vi "test_serial-w-arduino-1.vi"() -> ()   [LabVIEW 2019]
uses:
  <vilib>/Instr/_visa.llb/VISA Configure Serial Port (Instr).vi
panel:
  in  "s":bool
  in  "steer":u8(slide)=28 scale=15.0..35.0
  in  "dt":u32=50
  out "read buffer":string
  out "Numeric":i32
  out "Waveform Chart":u32(graph)
  in  "speed":u8(slide)=28 scale=1.0..255.0
  in  "write":bool
  in  "baud rate":u32=115200
  out "String":string
  in  "stop":bool
  out "write buffer":string
  in  "VISA resource name":refnum<visa-resource-name>="COM6"
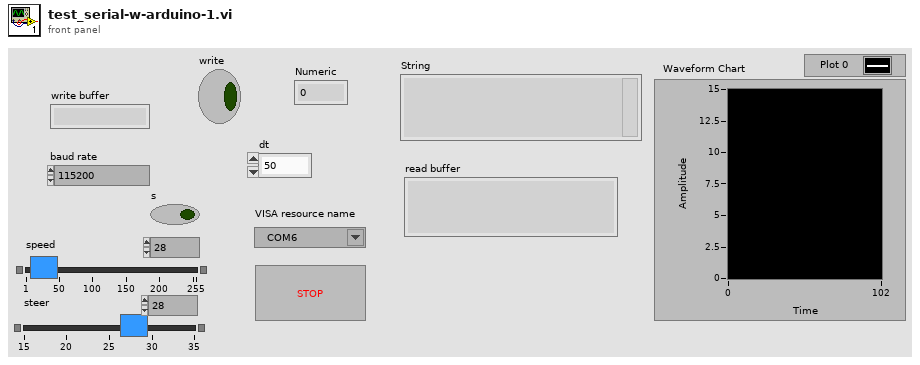
[diagram p1: front panel]
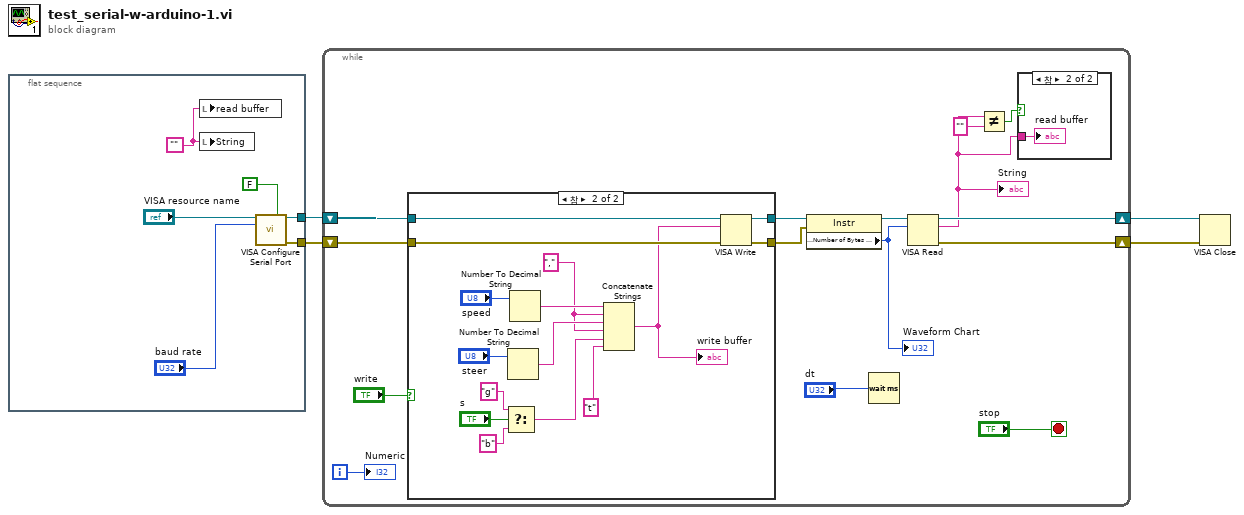
[diagram p0: block diagram]
diagram:
  n1 = flat-sequence {
    tunnel: [w9] -> w4
    tunnel: [w8] -> w1
    frame #0 {
      w5 = ""
      n2 = local write "read buffer"(w5) -> ()
      n3 = local write "String"(w5) -> ()
      n4 = call-poly "VISA Configure Serial Port"("VISA resource name"="VISA resource name", "Enable Termination\nChar (T)"=FALSE ("Enable Termination\nChar (T)"), "baud rate (9600)"="baud rate") -> ("VISA resource name out"=w9:refnum<visa-resource-name>, "error out"=w8:errorcluster)  [unwired: 11 in]
    }
  }
  n5 = while {
    shift-right: [w19] -> w3
    shift-left: w4 -> [w25]
    shift-right: [w16] -> w2
    shift-left: w1 -> [w24]
    i -> [w15]
    stop <- "stop" stop-if-true
    n6 = case shown="참" "write" {
      tunnel: w25 -> [w28 w43]
      tunnel: [w27 w42] -> w17
      tunnel: w24 -> [w27 w41]
      tunnel: [w28 w40] -> w20
      frame False {
      }
      frame True {
        w30 = "," ("string")
        n7 = Select(t="g" ("string"), s="s", f="b" ("string")) -> (s? t:f=w29:string)
        n8 = Number To Decimal String(number="steer") -> (decimal integer string=w34:string)  [unwired: 1 in]
        n9 = Number To Decimal String(number="speed") -> (decimal integer string=w38:string)  [unwired: 1 in]
        n10 = Concatenate Strings(w38, w30, w34, w30, w29, "t" ("string")) -> (w36:string)
        "write buffer" <- w36
        n11 = VISA Write(VISA resource name=w43, write buffer=w36, error in (no error)=w41) -> (VISA resource name out=w40:refnum<visa-resource-name>, error out=w42:errorcluster)  [unwired: 1 out]
      }
    }
    n12 = property class="Instr"(reference=w20, error in=w17) -> (reference out=w21:refnum<visa-resource-name>, "Serial Settings:Number of Bytes at Serial Port"=w14:u32)  [unwired: 1 out]
    "Waveform Chart" <- w14
    n13 = Wait (ms)(milliseconds to wait="dt") -> ()  [unwired: 1 out]
    n14 = VISA Read(VISA resource name=w21, byte count=w14) -> (VISA resource name out=w19:refnum<visa-resource-name>, read buffer=w11:string, error out=w16:errorcluster)  [unwired: 1 in, 1 out]
    "String" <- w11
    n15 = Not Equal?(x=w11, y="") -> (x != y?=w12:bool)
    n16 = case shown="참" w12 {
      tunnel: w11 -> [_ w26]
      frame False {
      }
      frame True {
        "read buffer" <- w26
      }
    }
    "Numeric" <- w15
  }
  n17 = VISA Close(VISA resource name=w3, error in (no error)=w2) -> ()  [unwired: 1 out]
